vi "FPGA_imu_gps.vi"() -> ()   [LabVIEW 2019]
uses:
  <vilib>/rvi/Emulation/niFpgaGetClockAttributes.vi
  <vilib>/rvi/Emulation/niFpgaSctlEmulationGetInTimedLoop.vi
  <vilib>/rvi/Emulation/niFpgaEmulationReportErrorSimple.vi
  <vilib>/rvi/Emulation/niFpgaCriticalErrorInLSC.vi
  Sub VIs/GPS/UART 8N1/UART 8N1 (FPGA).lvlib
panel:
  in  "Baud Rate":u32=9600
  out "Read Data":u8[](array[numeric])
  in  "Count(mSec)":u32
  out "SPI Read Acc Data":u8[](array[numeric])
  out "SPI Read Acc Config":u8[](array[numeric])
  out "SPI Read Gyro Config":u8[](array[numeric])
  out "SPI Read Gyro Data":u8[](array[numeric])
  out "SPI Read WHOAMI":u8[](array[numeric])
  # "UART"
  # "SPI"
  # "Gyroscope"
  # "WHOAMI"
  # "Accelerometer"
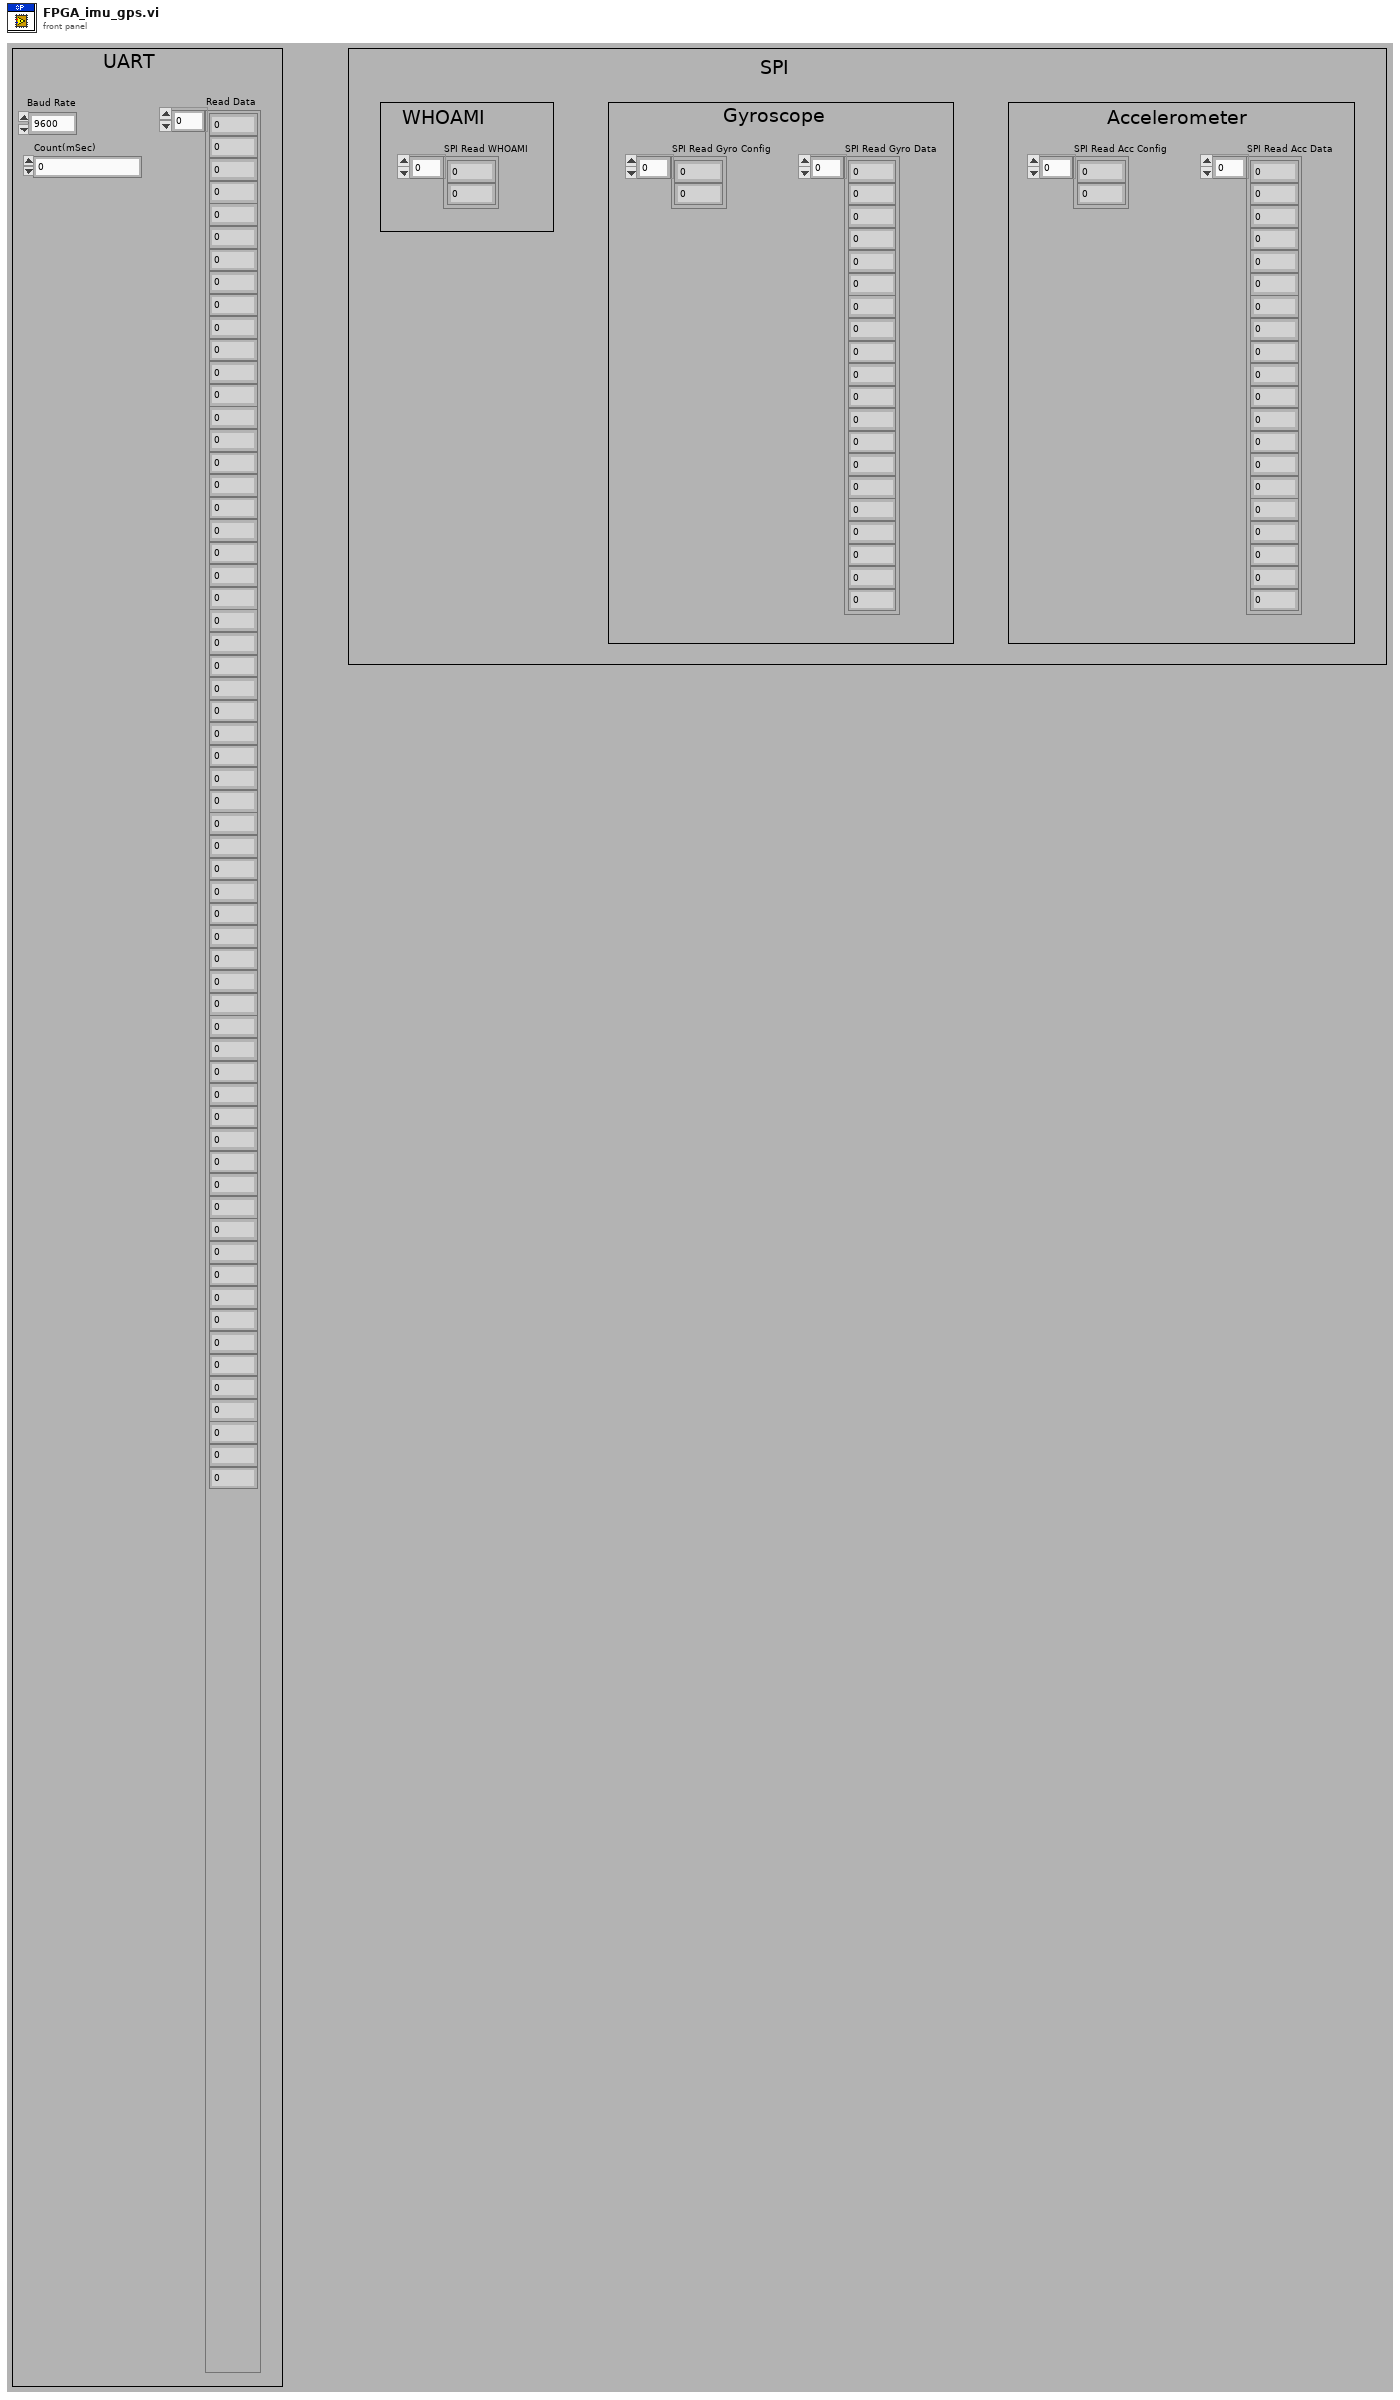
[diagram p1: front panel]
types:
  T1 = cluster{"SCLK":refnum<k21>, "CS":refnum<k21>, "MOSI":refnum<k21>, "MISO":refnum<k21>}
  T2 = typedef "UART 8N1 (FPGA).lvlib/UART Ref.ctl" = cluster{"FPGA I/O":refnum<k21>, "Buffer Ref":refnum<k21>, "Stop Ref":refnum<k21>}
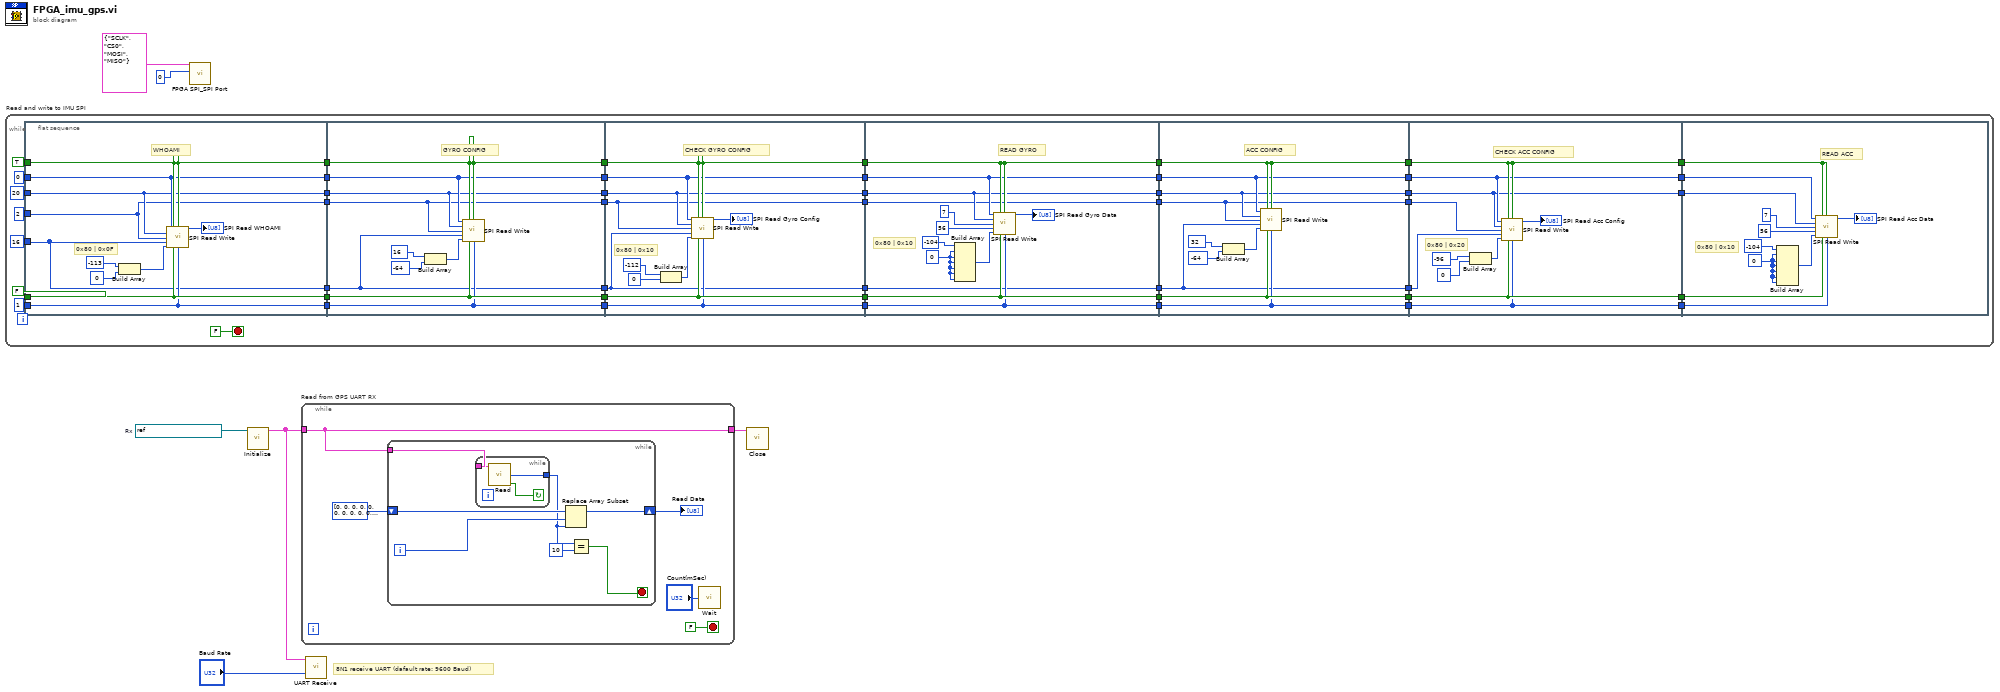
[diagram p0: block diagram]
diagram:
  w6 = refnum<k21> "ConnectorA/DIO0"  # Rx
  # "8N1 receive UART (dafault rate: 9600 Baud)"
  n1 = while "Read and write to IMU SPI" {
    stop <- FALSE stop-if-true
    n2 = flat-sequence {
      tunnel: i8 0 ("SPI_Port") -> [w63]
      tunnel: TRUE ("SPI_CPOL") -> [w64]
      tunnel: u32 20 ("SPI_Clock Divider") -> [w59]
      tunnel: u16 2 ("SPI_Total Bytes") -> [w58]
      tunnel: u16 16 ("SPI_Total Bits") -> [w57]
      tunnel: FALSE ("SPI_CS Active State") -> [w61]
      tunnel: u8 1 ("SPI_CS") -> [w60]
      tunnel: [w64] -> w49
      tunnel: [w63] -> w48
      tunnel: [w61] -> w45
      tunnel: [w60] -> w44
      tunnel: [w59] -> w43
      tunnel: [w58] -> w42
      tunnel: [w57] -> w41
      tunnel: w49 -> [w72]
      tunnel: w48 -> [w71]
      tunnel: w45 -> [w69]
      tunnel: w44 -> [w68]
      tunnel: w43 -> [w70]
      tunnel: w42 -> [w67]
      tunnel: w41 -> [w66]
      tunnel: [w72] -> w40
      tunnel: [w71] -> w38
      tunnel: [w70] -> w36
      tunnel: [w69] -> w34
      tunnel: [w68] -> w32
      tunnel: [w67] -> w30
      tunnel: [w66] -> w29
      tunnel: w40 -> [w84]
      tunnel: [w84] -> w39
      tunnel: w38 -> [w83]
      tunnel: [w83] -> w37
      tunnel: w36 -> [w80]
      tunnel: [w80] -> w35
      tunnel: w34 -> [w82]
      tunnel: [w82] -> w33
      tunnel: w32 -> [w81]
      tunnel: [w81] -> w31
      tunnel: w30 -> [w77]
      tunnel: w29 -> [w78]
      tunnel: [w78] -> w25
      tunnel: [w77] -> w20
      tunnel: w39 -> [w91]
      tunnel: w37 -> [w90]
      tunnel: w35 -> [w89]
      tunnel: w33 -> [w94]
      tunnel: w31 -> [w93]
      tunnel: [w94] -> w28
      tunnel: [w93] -> w27
      tunnel: w25 -> [w92]
      tunnel: [w92] -> w24
      tunnel: [w91] -> w23
      tunnel: [w90] -> w22
      tunnel: [w89] -> w21
      tunnel: w20 -> [w88]
      tunnel: [w88] -> w19
      tunnel: w28 -> [w103]
      tunnel: w27 -> [w102]
      tunnel: w24 -> [w100]
      tunnel: w23 -> [w106]
      tunnel: w22 -> [w105]
      tunnel: w21 -> [w104]
      tunnel: w19 -> [w101]
      tunnel: [w106] -> w18
      tunnel: [w105] -> w17
      tunnel: [w104] -> w16
      tunnel: [w103] -> w15
      tunnel: [w102] -> w14
      tunnel: [w101] -> w13
      tunnel: [w100] -> w12
      tunnel: w18 -> [w115]
      tunnel: w17 -> [w114]
      tunnel: w16 -> [w113]
      tunnel: w15 -> [w112]
      tunnel: w14 -> [w111]
      tunnel: w13 -> [w117]
      tunnel: w12 -> [w116]
      tunnel: [w115] -> w11
      tunnel: [w114] -> w10
      tunnel: [w113] -> w9
      tunnel: [w112] -> w8
      tunnel: [w111] -> w7
      tunnel: w11 -> [w126]
      tunnel: w10 -> [w125]
      tunnel: w9 -> [w124]
      tunnel: w8 -> [w123]
      tunnel: w7 -> [w122]
      frame #0 {
        # "0x80 | 0x0F"
        # "WHOAMI"
        n3 = Build Array(i8 -113 ("Port"), i8 0 ("Port")) -> (w62:i8[])
        n4 = call "SPI Read Write.vi"("SPI_Port"=w63, "SPI_CPOL"=w64, "SPI_CPHA"=w64, "SPI_Clock Divider"=w59, "SPI_Total Bytes"=w58, "SPI_Total Bits"=w57, "SPI_Write Data"=w62, "SPI_CS Active State"=w61, "SPI_CS"=w60) -> ("SPI_Read Data"=→"SPI Read WHOAMI":u8[])  [unwired: 6 in]
      }
      frame #1 {
        # "GYRO CONFIG"
        n5 = Build Array(i8 16 ("Port"), i8 -64 ("Port")) -> (w73:i8[])
        n6 = call "SPI Read Write.vi"("SPI_Port"=w71, "SPI_CPOL"=w72, "SPI_CPHA"=w72, "SPI_Clock Divider"=w70, "SPI_Total Bytes"=w67, "SPI_Total Bits"=w66, "SPI_Write Data"=w73, "SPI_CS Active State"=w69, "SPI_CS"=w68) -> ()  [unwired: 6 in, 1 out]
      }
      frame #2 {
        # "0x80 | 0x10"
        # "CHECK GYRO CONFIG"
        n7 = Build Array(i8 -112 ("Port"), i8 0 ("Port")) -> (w86:i8[])
        n8 = call "SPI Read Write.vi"("SPI_Port"=w83, "SPI_CPOL"=w84, "SPI_CPHA"=w84, "SPI_Clock Divider"=w80, "SPI_Total Bytes"=w77, "SPI_Total Bits"=w78, "SPI_Write Data"=w86, "SPI_CS Active State"=w82, "SPI_CS"=w81) -> ("SPI_Read Data"=→"SPI Read Gyro Config":u8[])  [unwired: 6 in]
      }
      frame #3 {
        w98 = i8 0 ("Port")
        # "0x80 | 0x10"
        # "READ GYRO"
        n9 = Build Array(i8 -104 ("Port"), w98, w98, w98, w98, w98, w98) -> (w99:i8[])
        n10 = call "SPI Read Write.vi"("SPI_Port"=w90, "SPI_CPOL"=w91, "SPI_CPHA"=w91, "SPI_Clock Divider"=w89, "SPI_Total Bytes"=u16 7, "SPI_Total Bits"=u16 56, "SPI_Write Data"=w99, "SPI_CS Active State"=w94, "SPI_CS"=w93) -> ("SPI_Read Data"=→"SPI Read Gyro Data":u8[])  [unwired: 6 in]
      }
      frame #4 {
        # "ACC CONFIG"
        n11 = Build Array(i8 32 ("Port"), i8 -64 ("Port")) -> (w107:i8[])
        n12 = call "SPI Read Write.vi"("SPI_Port"=w105, "SPI_CPOL"=w106, "SPI_CPHA"=w106, "SPI_Clock Divider"=w104, "SPI_Total Bytes"=w101, "SPI_Total Bits"=w100, "SPI_Write Data"=w107, "SPI_CS Active State"=w103, "SPI_CS"=w102) -> ()  [unwired: 6 in, 1 out]
      }
      frame #5 {
        # "0x80 | 0x20"
        # "CHECK ACC CONFIG"
        n13 = Build Array(i8 -96 ("Port"), i8 0 ("Port")) -> (w120:i8[])
        n14 = call "SPI Read Write.vi"("SPI_Port"=w114, "SPI_CPOL"=w115, "SPI_CPHA"=w115, "SPI_Clock Divider"=w113, "SPI_Total Bytes"=w117, "SPI_Total Bits"=w116, "SPI_Write Data"=w120, "SPI_CS Active State"=w112, "SPI_CS"=w111) -> ("SPI_Read Data"=→"SPI Read Acc Config":u8[])  [unwired: 6 in]
      }
      frame #6 {
        w128 = i8 0 ("Port")
        # "0x80 | 0x10"
        # "READ ACC"
        n15 = Build Array(i8 -104 ("Port"), w128, w128, w128, w128, w128, w128) -> (w127:i8[])
        n16 = call "SPI Read Write.vi"("SPI_Port"=w125, "SPI_CPOL"=w126, "SPI_CPHA"=w126, "SPI_Clock Divider"=w124, "SPI_Total Bytes"=u16 7, "SPI_Total Bits"=u16 56, "SPI_Write Data"=w127, "SPI_CS Active State"=w123, "SPI_CS"=w122) -> ("SPI_Read Data"=→"SPI Read Acc Data":u8[])  [unwired: 6 in]
      }
    }
  }
  n17 = call "FPGA SPI_SPI Port.vi"("Port"=i8 0, "FPGA IO"=T1 {"SCLK"="SCLK", "CS"="CS0", "MOSI"="MOSI", "MISO"="MISO"}) -> ()  [unwired: 10 out]
  n18 = call "Initialize.vi"("FPGA I/O"=w6) -> ("BPT Ref"=w4:T2)  [unwired: 14 in]
  n19 = while "Read from GPS UART RX" {
    tunnel: [w136] -> w5
    tunnel: w4 -> [w136]
    stop <- FALSE stop-if-true
    n20 = while {
      tunnel: w136 -> [w143]
      shift-right: [w139] -> w135
      shift-left: u8[] [0, 0, 0, 0, 0, 0, 0, 0, 0, 0, 0, 0, 0, 0, 0, 0, 0, 0, 0, 0, 0, 0, 0, 0, 0, 0, 0, 0, 0, 0, 0, 0, 0, 0, 0, 0, 0, 0, 0, 0, 0, 0, 0, 0, 0, 0, 0, 0, 0, 0, 0, 0, 0, 0, 0, 0, 0, 0, 0, 0, 0, 0, 0, 0, 0, 0, 0, 0, 0, 0, 0, 0, 0, 0, 0, 0, 0, 0, 0, 0, 0, 0, 0, 0, 0, 0, 0, 0, 0, 0, 0, 0, 0, 0, 0, 0, 0, 0, 0, 0] ("array") -> [w140]
      i -> [w141]
      stop <- w137 stop-if-true
      n21 = while {
        tunnel: w143 -> [w146]
        tunnel: [w145] -> w138
        stop <- w144 continue-if-true
        n22 = call "Read.vi"("UART Ref In"=w146) -> ("Data"=w145:u8, "Timed Out?"=w144:bool)  [unwired: 12 in, 1 out]
      }
      n23 = Replace Array Subset(array=w140, new element=w138, index=w141) -> (w139:u8[])
      n24 = Equal?(x=w138, y=u8 10) -> (x = y?=w137:bool)
    }
    "Read Data" <- w135
    n25 = call "Wait"("Count(mSec)"="Count(mSec)") -> ()  [unwired: 1 out]
  }
  n26 = call "UART Receive.vi"("UART Ref"=w4, "Baud Rate (9600)"="Baud Rate") -> ()  [unwired: 14 in]
  n27 = call "Close.vi"("UART Ref"=w5) -> ()  [unwired: 15 in]
